vi "MAIN_Shut_down.vi"(3 "queue FPGA":refnum<queue>, 4 "Q_pump":refnum<queue>, 5 "Start acquisition":bool, 6 "Q_valve":refnum<queue>, 7 "Q_DAQ":refnum<queue>, 8 "error in":errorcluster, 9 "Q_CAMERA":refnum<queue>, 10 "Q_ASI":refnum<queue>, 11 "Q_piezo":refnum<queue>) -> (0 "error out":errorcluster)   [LabVIEW 2015]
uses:
  CONTROLS/Q_MCL_piezo_element.ctl
  CONTROLS/Q_ASI_stage_element.ctl
  CONTROLS/Q_DAQ_element.ctl
  CONTROLS/Q_camera_element.ctl
  CONTROLS/Q_VALVE_element.ctl
  CONTROLS/Q_PUMP_element.ctl
  CONTROLS/Q_FPGA_element.ctl
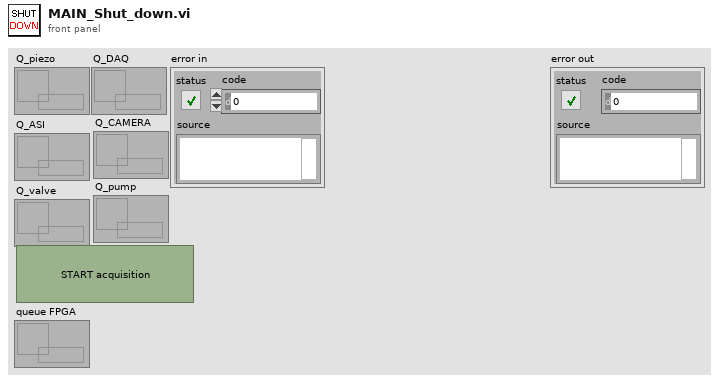
[diagram p1: front panel]
types:
  T1 = typedef "Q_FPGA_element.ctl" = cluster{"variant":variant, "Instruction":enum16{"FPGA_idle", "FPGA_initialize", "FPGA_error", "FPGA_security_stop", "FPGA_laser", "FPGA_start_stop_measure_QPD", "FPGA_measure_QPD", "FPGA_measure_QPD_noise", "FPGA_stop_measure_QPD", "FPGA_init_autofocus", "FPGA_init_single_scan", "FPGA_stop_single_scan", "FPGA_init_merFISH", "FPGA_measure_QPD_merFISH", "FPGA_init_scan_merFISH", "FPGA_scan_merFISH", "FPGA_close_merFISH", "FPGA_stop"}}
  T2 = typedef "Q_PUMP_element.ctl" = cluster{"variant":variant, "Instruction":enum16{"PUMP_idle", "PUMP_initialize", "PUMP_error", "PUMP_security_stop", "PUMP_read_pressure", "PUMP_change_pressure", "PUMP_init_merFISH", "PUMP_change_presure_merFISH", "PUMP_zero_pressure_merFISH", "PUMP_close_merFISH", "PUMP_stop"}}
  T3 = typedef "Q_VALVE_element.ctl" = cluster{"variant":variant, "Instruction":enum16{"VALVE_idle", "VALVE_initialize", "VALVE_error", "VALVE_security_stop", "VALVE_change_position", "VALVE_two_way_valves", "VALVE_init_merFISH", "VALVE_stop"}}
  T4 = typedef "Q_DAQ_element.ctl" = cluster{"variant":variant, "Instruction":enum16{"DAQ_idle", "DAQ_initialize", "DAQ_error", "DAQ_security_stop", "DAQ_init_single_scan", "DAQ_single_scan", "DAQ_init_merFISH", "DAQ_scan_merFISH", "DAQ_photobleaching_merFISH", "DAQ_close_merFISH", "DAQ_stop"}}
  T5 = typedef "Q_MCL_piezo_element.ctl" = cluster{"variant":variant, "Instruction":enum16{"Piezo_idle", "Piezo_initialize", "Piezo_error", "Piezo_security_stop", "Piezo_read_z", "Piezo_move_z", "Piezo_keyboard_move", "Piezo_close_autofocus_calibration_ramp", "Piezo_change_init_state", "Piezo_init_autofocus", "Piezo_init_autofocus_merFISH_TL", "Piezo_autofocus", "Piezo_autofocus_merFISH_TL", "Piezo_stop_autofocus", "Piezo_stop_autofocus_merFISH_TL", "Piezo_autofocus_lost", "Piezo_resume_autofocus_merFISH_TL", "Piezo_check_z_position_merFISH_TL", "Piezo_init_ramp", "Piezo_move_z_ramp", "Piezo_close_ramp", "Piezo_close_merFISH", "Piezo_stop"}}
  T6 = typedef "Q_ASI_stage_element.ctl" = cluster{"variant":variant, "Instruction":enum16{"ASI_idle", "ASI_initialize", "ASI_error", "ASI_security_stop", "ASI_read_XYZ", "ASI_up", "ASI_down", "ASI_left", "ASI_right", "ASI_save_XY", "ASI_move_to_XY", "ASI_brightfield", "ASI_init_scan", "ASI_init_merFISH", "ASI_move_to_XY_merFISH", "ASI_move_to_Z_merFISH", "ASI_init_autofocus_search_merFISH", "ASI_close_autofocus_search_merFISH", "ASI_adjust_piezo_autofocus_merFISH", "ASI_set_piezo_autofocus_to_reference_position_merFISH_TL", "ASI_close_merFISH", "ASI_stop"}}
  T7 = typedef "Q_camera_element.ctl" = cluster{"variant":variant, "Instruction":enum16{"CAMERA_idle", "CAMERA_initialize", "CAMERA_error", "CAMERA_security_stop", "CAMERA_not_acquiring", "CAMERA_acquiring", "CAMERA_start_acquiring", "CAMERA_stop_acquiring", "CAMERA_change_exposure", "CAMERA_define_ROI", "CAMERA_cooler", "CAMERA_acquire_movie", "CAMERA_init_scan", "CAMERA_check_image_scan", "CAMERA_close_scan", "CAMERA_init_merFISH", "CAMERA_start_acquiring_merFISH", "CAMERA_close_scan_merFISH", "CAMERA_close_merFISH", "CAMERA_STOP"}}
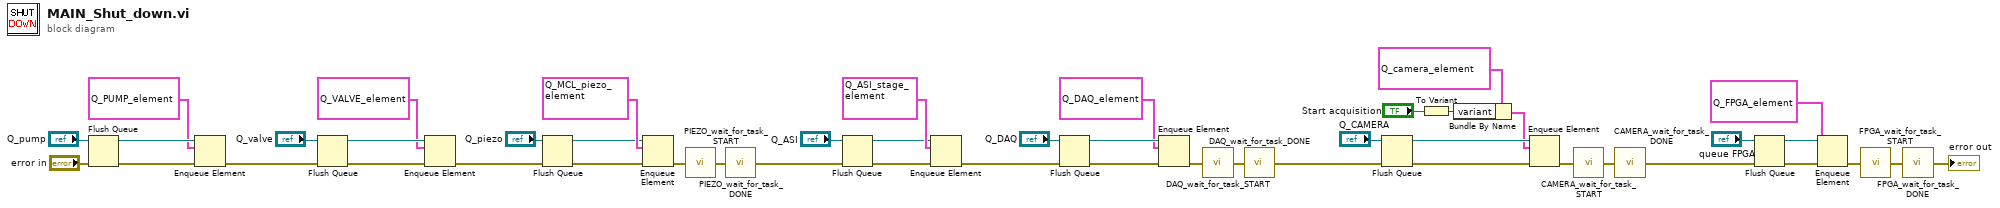
[diagram p0: block diagram]
diagram:
  n1 = Flush Queue(queue="Q_pump", error in (no error)="error in") -> (queue out=w25:refnum<queue>, error out=w22:errorcluster)  [unwired: 1 out]
  n2 = Enqueue Element(queue=w25, element=T2 {"variant"=variant, "Instruction"=enum."PUMP_stop"} ("Q_PUMP"), error in (no error)=w22) -> (error out=w20:errorcluster)  [unwired: 1 in, 2 out]
  n3 = Flush Queue(queue="Q_valve", error in (no error)=w20) -> (queue out=w29:refnum<queue>, error out=w24:errorcluster)  [unwired: 1 out]
  n4 = Enqueue Element(queue=w29, element=T3 {"variant"=variant, "Instruction"=enum."VALVE_stop"} ("Q_VALVE"), error in (no error)=w24) -> (error out=w27:errorcluster)  [unwired: 1 in, 2 out]
  n5 = Flush Queue(queue="Q_piezo", error in (no error)=w27) -> (queue out=w44:refnum<queue>, error out=w43:errorcluster)  [unwired: 1 out]
  n6 = Enqueue Element(queue=w44, element=T5 {"variant"=variant, "Instruction"=enum."Piezo_stop"} ("Q_MCL_Piezo"), error in (no error)=w43) -> (error out=w19:errorcluster)  [unwired: 1 in, 2 out]
  n7 = call "PIEZO_wait_for_task_START.vi"("error in"=w19) -> ("error out"=w18:errorcluster)
  n8 = call "PIEZO_wait_for_task_DONE.vi"("error in"=w18) -> ("error out"=w17:errorcluster)
  n9 = Flush Queue(queue="Q_ASI", error in (no error)=w17) -> (queue out=w40:refnum<queue>, error out=w41:errorcluster)  [unwired: 1 out]
  n10 = Enqueue Element(queue=w40, element=T6 {"variant"=variant, "Instruction"=enum."ASI_stop"}, error in (no error)=w41) -> (error out=w32:errorcluster)  [unwired: 1 in, 2 out]
  n11 = Flush Queue(queue="Q_DAQ", error in (no error)=w32) -> (queue out=w47:refnum<queue>, error out=w46:errorcluster)  [unwired: 1 out]
  n12 = Enqueue Element(queue=w47, element=T4 {"variant"=variant, "Instruction"=enum."DAQ_stop"} ("Q_DAQ"), error in (no error)=w46) -> (error out=w1:errorcluster)  [unwired: 1 in, 2 out]
  n13 = call "DAQ_wait_for_task_START.vi"("error in"=w1) -> ("error out"=w16:errorcluster)
  n14 = call "DAQ_wait_for_task_DONE.vi"("error in"=w16) -> ("error out"=w15:errorcluster)
  n15 = Flush Queue(queue="Q_CAMERA", error in (no error)=w15) -> (queue out=w37:refnum<queue>, error out=w36:errorcluster)  [unwired: 1 out]
  n16 = To Variant(anything="Start acquisition") -> (Variant=w12:variant)
  n17 = Bundle By Name(cluster=T7 {"variant"=variant, "Instruction"=enum."CAMERA_STOP"} ("Q_ANDOR_element"), "variant"=w12) -> (w11:T7)
  n18 = Enqueue Element(queue=w37, element=w11, error in (no error)=w36) -> (error out=w39:errorcluster)  [unwired: 1 in, 2 out]
  n19 = call "CAMERA_wait_for_task_START.vi"("error in"=w39) -> ("error out"=w38:errorcluster)
  n20 = call "CAMERA_wait_for_task_DONE.vi"("error in"=w38) -> ("error out"=w9:errorcluster)
  n21 = Flush Queue(queue="queue FPGA", error in (no error)=w9) -> (queue out=w6:refnum<queue>, error out=w7:errorcluster)  [unwired: 1 out]
  n22 = Enqueue Element(queue=w6, element=T1 {"variant"=variant, "Instruction"=enum."FPGA_stop"}, error in (no error)=w7) -> (error out=w4:errorcluster)  [unwired: 1 in, 2 out]
  n23 = call "FPGA_wait_for_task_START.vi"("error in"=w4) -> ("error out"=w3:errorcluster)
  n24 = call "FPGA_wait_for_task_DONE.vi"("error in"=w3) -> ("error out"=→"error out":errorcluster)
